vi "ElevatorSim_GetCurrentDraw.vi"(11 "ElevatorSim":T1 {"GearBox"."Kt_NMPerAmp" format="%13.5p"; "GearBox"."Kv_RadPerSecPerVolt" format="%13.5p"; "GearBox"."R_Ohms" format="%13.5p"; "GearBox"."FreeSpeed_RadPerSec" format="%13.5p"; "GearBox"."FreeCurrent_Amps" format="%13.5p"; "GearBox"."StallCurrent_Amps" format="%13.5p"; "GearBox"."StallTorque_NM" format="%13.5p"; "GearBox"."nominalVoltage_Volts" format="%13.5p"}) -> (3 "Current_Amps":dbl)   [LabVIEW 2019, in "Trajectory_Library.lvlib"]
doc: "Creates a new LINEAR SYSTEM data cluster with the specified values. \n\n\nInputs: \n - XXX -- XXX.\n\nOutputs:\n - XXX -- XXX."
uses:
  Trajectory_Library.lvlib
  ELEVATOR_SIM.ctl
  LINEAR_SYSTEM_SIM.ctl
  LINEAR_SYSTEM.ctl
  <vilib>/Analysis/Matrix/Datatypes/RealMatrix.ctl
  DCMOTOR.CTL
  <vilib>/Analysis/Matrix/NI_Matrix.lvlib
panel:
  # "<States, 1>"
  # "<Outputs, 1>"
  # "<Inputs, 1>"
  # "<Outputs, 1>"
  # "<States,States>"
  # "<States,Inputs>"
  # "<Outputs,States>"
  # "<Outputs,Inputs>"
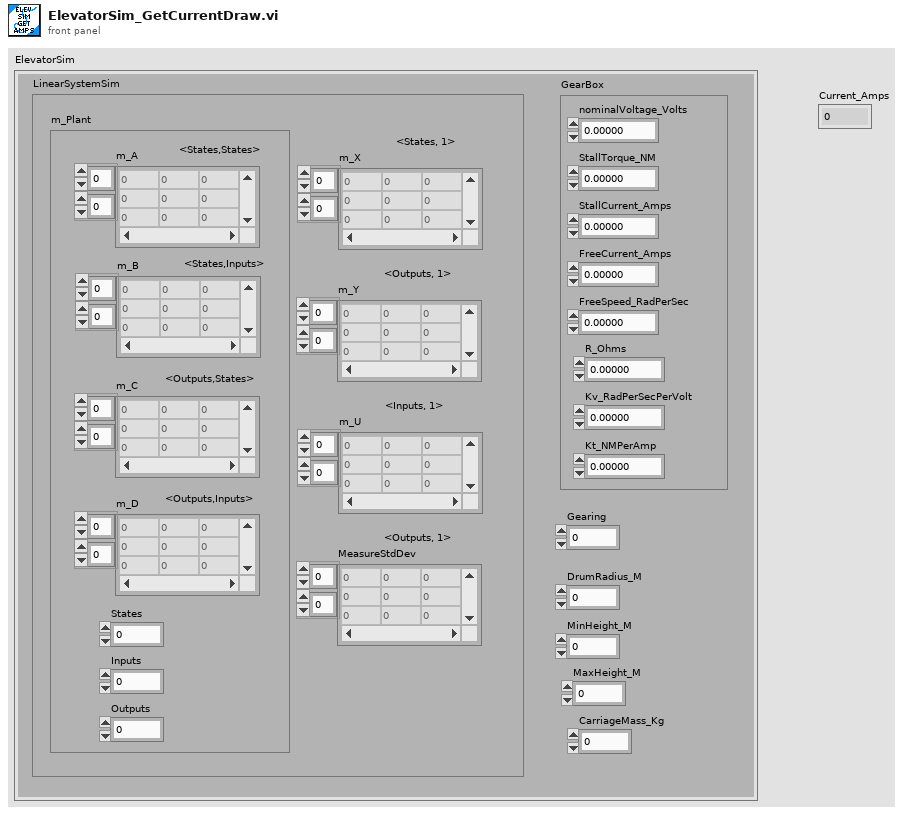
[diagram p1: front panel]
types:
  T1 = typedef "Trajectory_Library.lvlib/ELEVATOR_SIM.ctl" = cluster{"LinearSystemSim":T2, "GearBox":T5, "Gearing":dbl, "DrumRadius_M":dbl, "MinHeight_M":dbl, "MaxHeight_M":dbl, "CarriageMass_Kg":dbl}
  T2 = typedef "Trajectory_Library.lvlib/LINEAR_SYSTEM_SIM.ctl" = cluster{"m_Plant":T3, "m_X":T4, "m_Y":T4, "m_U":T4, "MeasureStdDev":T4}
  T3 = typedef "Trajectory_Library.lvlib/LINEAR_SYSTEM.ctl" = cluster{"m_A":T4, "m_B":T4, "m_C":T4, "m_D":T4, "States":i32, "Inputs":i32, "Outputs":i32}
  T4 = typedef "NI_Matrix.lvlib/RealMatrix.ctl" = dbl[][]
  T5 = typedef "Trajectory_Library.lvlib/DCMOTOR.CTL" = cluster{"nominalVoltage_Volts":dbl, "StallTorque_NM":dbl, "StallCurrent_Amps":dbl, "FreeCurrent_Amps":dbl, "FreeSpeed_RadPerSec":dbl, "R_Ohms":dbl, "Kv_RadPerSecPerVolt":dbl, "Kt_NMPerAmp":dbl}
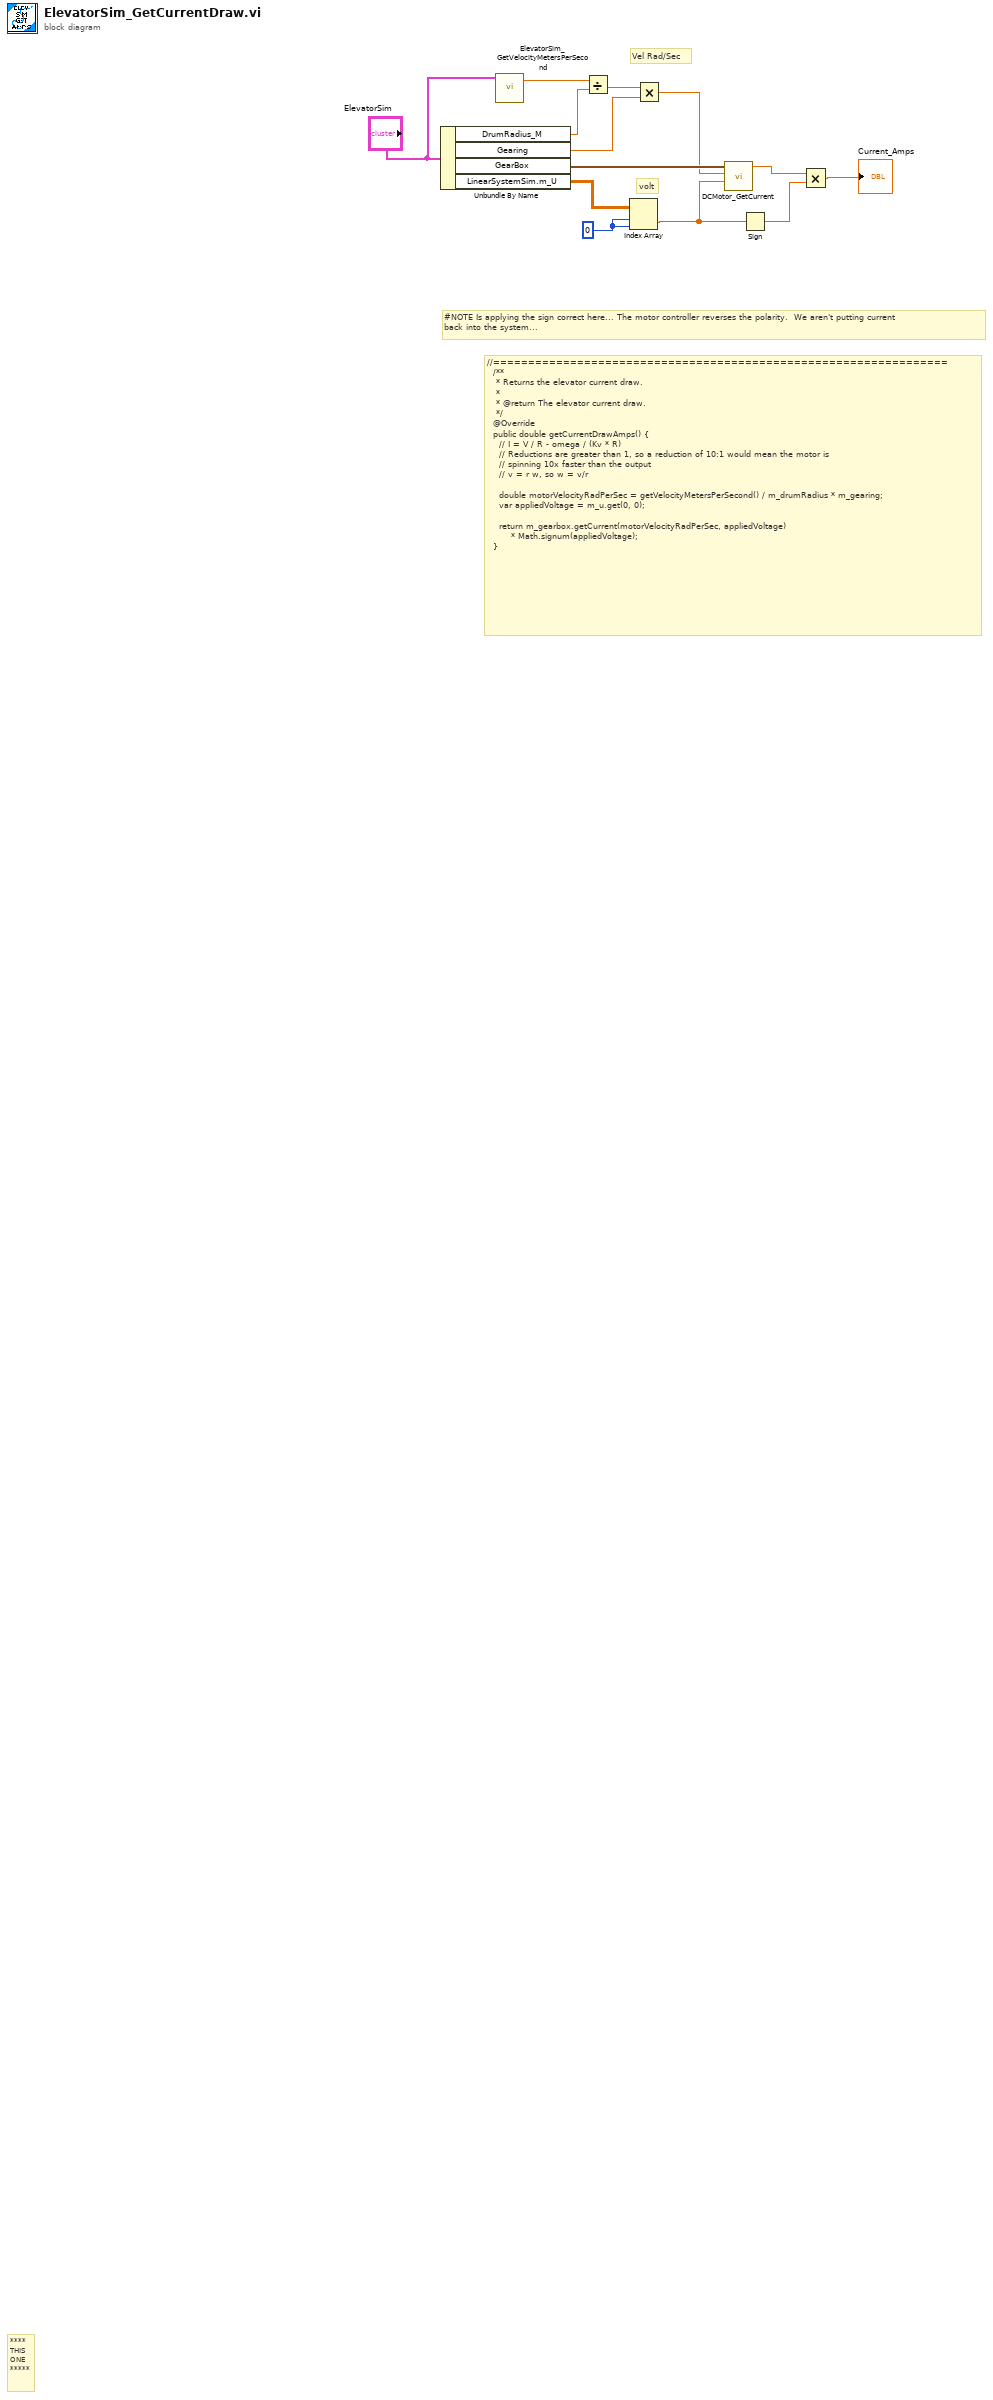
[diagram p0: block diagram]
diagram:
  w8 = 0 ("index (row)")
  # "#NOTE Is applying the sign correct here... The motor controller reverses the polarity.  We aren't putting current\nback into the system..."
  # "volt"
  # "Vel Rad/Sec"
  # "//=================================================================\n  /**\n   * Returns the elevator current draw.\n   *\n   * @return The elevator current draw.\n   */\n  @Override\n  public double getCurrentDrawAmps() {\n    // I = V / R - omega / (Kv * R)\n    // Reductions are greater than 1, so a reduction of 10:1 would mean the motor is\n    // spinning 10x faster than the output\n    // v = r w, so w = v/r\n\n    double motorVelocityRadPerSec = getVelocityMetersPerSecond() / m_drumRadius * m_gearing;\n    var appliedVoltage = m_u.get(0, 0);\n\n    return m_gearbox.getCurrent(motorVelocityRadPerSec, appliedVoltage)\n        * Math.signum(appliedVoltage);\n  }"
  # "****\nTHIS\nONE\n*****"
  n1 = Unbundle By Name("ElevatorSim") -> ("DrumRadius_M"=w11:dbl, "Gearing"=w9:dbl, "GearBox"=w6:T5, "LinearSystemSim.m_U"=w7:T4)
  n2 = call "ElevatorSim_GetVelocityMetersPerSecond.vi"("ElevatorSim"="ElevatorSim") -> ("Velocity_MetersPerSec"=w12:dbl)  [unwired: 10 in]
  n3 = Divide(x=w12, y=w11) -> (x/y=w10:dbl)
  n4 = Index Array(array=w7, index (row)=w8, index (col)=w8) -> (element=w4:dbl)
  n5 = Multiply(x=w10, y=w9) -> (x*y=w5:dbl)
  n6 = call "DCMotor_GetCurrent.vi"("VoltageInput_Volts"=w4, "Speed_RadPerSec"=w5, "DCMOTOR"=w6) -> ("Current_Amps"=w3:dbl)  [unwired: 8 in]
  n7 = Sign(1:w4) -> (0:w2:dbl)
  n8 = Multiply(x=w3, y=w2) -> (x*y=→"Current_Amps":dbl)
